vi "Stop Core.vi"(10 "final error code":i32, 11 "TestSinWaveProc in":refnum<class "TestSinWaveProc.lvclass">) -> (3 "TestSinWaveProc out":refnum<class "TestSinWaveProc.lvclass">)   [LabVIEW 2024, in "TestSinWaveActor.lvlib" / "TestSinWaveProc.lvclass"]
doc: "(<B>Filename</B>: Actor Framework.lvlib:Actor.lvclass:Stop Core.vi)\n\nDefines what the actor does before it stops. Use the <B>final error code</B> input to determine whether the actor shut down in response to an error.\n\nBy default, this method does nothing. A descendant class may override it to define behavior, such as shutting down any processes the actor initiated in its override of the Actor Core method."
uses:
  TestSinWaveProc.lvclass
  TestSinWaveProc.lvclass/TestSinWaveProc.ctl
  <vilib>/ActorFramework/Actor/Actor.lvclass
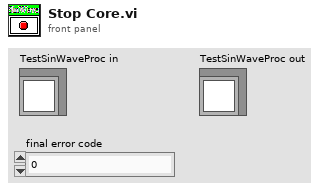
[diagram p1: front panel]
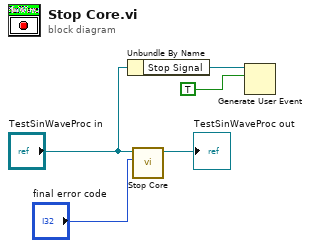
[diagram p0: block diagram]
diagram:
  n1 = Unbundle By Name("TestSinWaveProc in") -> ("Stop Signal"=w2:refnum<user-event>)
  n2 = call-parent "Stop Core.vi"("final error code"="final error code", "Actor in"="TestSinWaveProc in") -> ("Actor out"=→"TestSinWaveProc out":refnum<class "TestSinWaveProc.lvclass">)  [unwired: 9 in]
  n3 = Generate User Event(user event=w2, event data cluster=TRUE) -> ()  [unwired: 2 in, 2 out]
